vi "Inst.Krohn-Hite-7008.GetPublicEvents.vi"(8 "error in (no error)":errorcluster, 11 "Inst.Krohn-Hite-7008 in":refnum<class "Inst.Krohn-Hite-7008.lvclass">) -> (0 "error out":errorcluster, 2 "Inst.Krohn-Hite-7008 Public Events":T1, 3 "Inst.Krohn-Hite-7008 out":refnum<class "Inst.Krohn-Hite-7008.lvclass">)   [LabVIEW 2019, in "Inst.Krohn-Hite-7008.lvclass"]
uses:
  Inst.Krohn-Hite-7008.lvclass
  <userlib>/LevyLab/Instrument Framework/SMOs/RemoteControl/Typedefs/Message--Cluster.ctl
  <userlib>/LevyLab/Instrument Framework/SMOs/RemoteControl/RemoteControl.lvclass
  Typedefs/PublicEvents--Inst.Krohn-Hite-7008.MessageFromProcess.ctl
  Typedefs/PublicEvents--Cluster.ctl
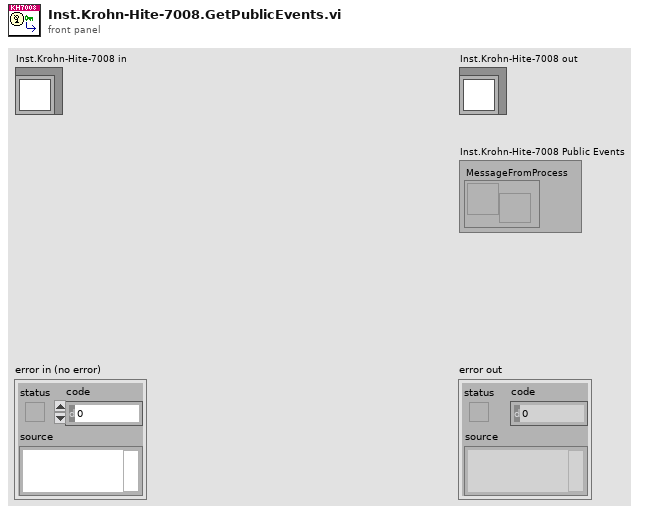
[diagram p1: front panel]
types:
  T1 = typedef "Inst.Krohn-Hite-7008.lvclass/PublicEvents--Cluster.ctl" = cluster{"MessageFromProcess":refnum<user-event>}
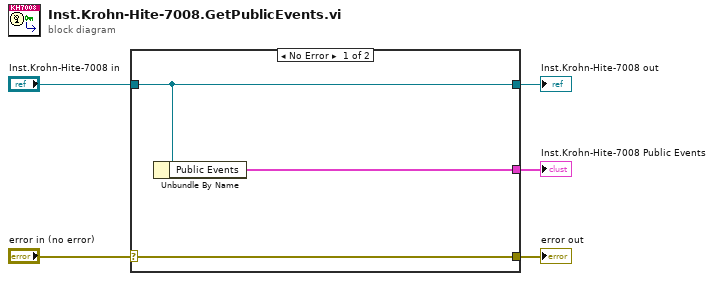
[diagram p0: block diagram]
diagram:
  n1 = case shown="No Error" "error in (no error)" {
    selector: "error in (no error)" -> [w8 w9]
    tunnel: [w8 w9] -> w4
    tunnel: [w7 w10] -> w2
    tunnel: "Inst.Krohn-Hite-7008 in" -> [w7 w10]
    tunnel: [w6 _] -> w1
    frame No Error {
      n2 = Unbundle By Name(w7) -> ("Public Events"=w6:T1)
    }
    frame Error {
    }
  }
  "error out" <- w4
  "Inst.Krohn-Hite-7008 out" <- w2
  "Inst.Krohn-Hite-7008 Public Events" <- w1
